vi "Get.vi"(10 "Index":i32, 11 "Variables in":refnum<class "Variables.lvclass">) -> (2 "Value":dbl)   [LabVIEW 2020, in "VolatusSeq.lvlib" / "Variables.lvclass"]
uses:
  Variables.lvclass
  Variables.lvclass/Variables.ctl
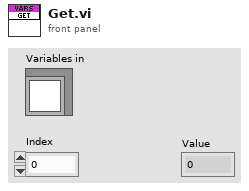
[diagram p1: front panel]
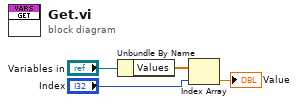
[diagram p0: block diagram]
diagram:
  n1 = Unbundle By Name("Variables in") -> ("Values"=w3:dbl[])
  n2 = Index Array(array=w3, index="Index") -> (element=→"Value":dbl)
